vi "FA Bending View.vi"() -> ()   [LabVIEW 2016, in "M1M3SupportEUI_Views.lvlib"]
uses:
  M1M3SupportEUI_Views.lvlib
  Model/Model.lvclass
  M1M3 Support Events/M1M3 Support Events.lvclass/M1M3 Support Events.ctl
  SALLV_m1m3/DataTypes/command_ApplyAberrationForcesByBendingModes.ctl
  SALLV_m1m3/DataTypes/command_ClearAberrationForces.ctl
  SALLV_m1m3/DataTypes/command_ApplyActiveOpticForcesByBendingModes.ctl
  SALLV_m1m3/DataTypes/command_ClearActiveOpticForces.ctl
  M1M3 Support Events/M1M3 Support Events.lvclass
  SALLV_m1m3/SALLV_m1m3.lvlib
  EUI Events/EUI Events.lvclass
panel:
  in  "ClearActiveOpticsButton":bool
  in  "ApplyActiveOpticsByBendingModesButton":bool
  in  "ClearAberrationButton":bool
  in  "ApplyAberrationByBendingModesButton":bool
  in  "Model in":refnum<class "Model.lvclass">
  in  "BM1":sgl
  in  "BM2":sgl
  in  "BM3":sgl
  in  "BM4":sgl
  in  "BM5":sgl
  in  "BM6":sgl
  in  "BM7":sgl
  in  "BM8":sgl
  in  "BM9":sgl
  in  "BM20":sgl
  in  "BM10":sgl
  in  "BM12":sgl
  in  "BM13":sgl
  in  "BM14":sgl
  in  "BM15":sgl
  in  "BM16":sgl
  in  "BM17":sgl
  in  "BM18":sgl
  in  "BM19":sgl
  in  "BM11":sgl
  in  "BM22":sgl
  in  "BM21":sgl
  # "Force Actuator\nApply/Clear Bending Modes"
  # "Bending Modes"
  # "0"
  # "1"
  # "2"
  # "3"
  # "4"
  # "5"
  # "6"
  # "7"
  # "8"
  # "9"
  # "00"
  # "10"
  # "20"
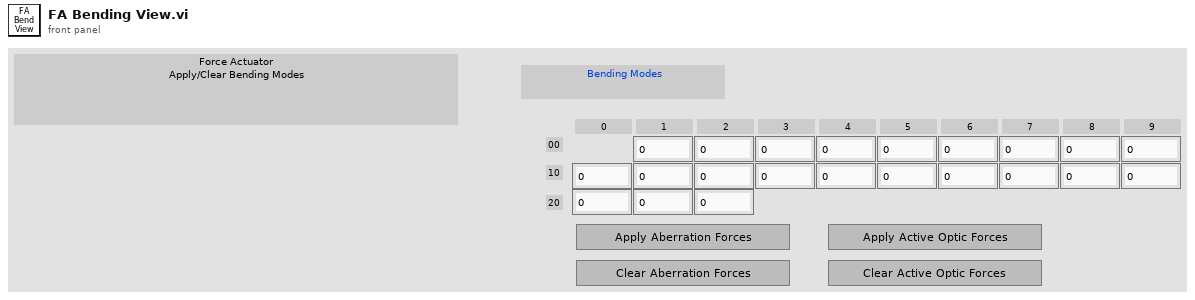
[diagram p1: front panel]
types:
  T1 = typedef "M1M3SupportEUI_TypeDefs.lvlib/M1M3 Support Events.ctl" = cluster{"Inclinometer  Data":refnum<user-event>, "IMS Data":refnum<user-event>, "SAL Connected":refnum<user-event>, "Accelerometer Data":refnum<user-event>, "OuterLoop Data":refnum<user-event>, "ErrorCode Event":refnum<user-event>, "InterlockStatus Event":refnum<user-event>, "InterlockWarning Event":refnum<user-event>, "Gyro Data":refnum<user-event>, "HP Actuator Info Event":refnum<user-event>, " FA Info Event":refnum<user-event>, "HP Monitor Info Event":refnum<user-event>, "FA Data":refnum<user-event>, "HP Actuator data":refnum<user-event>, "HP Monitor data":refnum<user-event>, "Air Supply Status Event":refnum<user-event>, "Air Supply Warning Event":refnum<user-event>, "Power Data":refnum<user-event>, "PID Data":refnum<user-event>, "PID Info Event":refnum<user-event>, "Power Status Event":refnum<user-event>, "Power Supply Status Event":refnum<user-event>, "Power Warning Event":refnum<user-event>, "Summary State Event":refnum<user-event>, "Detailed State Event":refnum<user-event>, "FA Force Warning Event":refnum<user-event>, "FA Warning Event":refnum<user-event>, "FA State Event":refnum<user-event>, "Applied AberrationForces Event":refnum<user-event>, "Applied Acceleration Forcces Event":refnum<user-event>, "Applied Azimuth Forces Event":refnum<user-event>, "Applied Active Optic Forces Event":refnum<user-event>, "Applied Balance Forces Event":refnum<user-event>, "Applied Cylinder Forces Event":refnum<user-event>, "Applied Elevation Forces Event":refnum<user-event>, "Applied Forces Event":refnum<user-event>, "Applied Offset Forces Event":refnum<user-event>, "Applied Static Forces Event":refnum<user-event>, "Applied Thermal Forces Event":refnum<user-event>, "Applied Velocity Forces Event":refnum<user-event>, "Rejected Aberration Force Event":refnum<user-event>, "Rejected Acceleration Forces Event":refnum<user-event>, "Rejected Active Optic Forces Event":refnum<user-event>, "Rejected Azimuth Forces Event":refnum<user-event>, "Rejected Balance Forces Event":refnum<user-event>, "Rejected Cylinder Forces Event":refnum<user-event>, "Rejected Elevation Forces Event":refnum<user-event>, "Rejected Forces Event":refnum<user-event>, "Rejected Offset Forces Event":refnum<user-event>, "Rejected Static Forces Event":refnum<user-event>, "Rejected Thermal Forces Event":refnum<user-event>, "Rejected Velocity Forces Event":refnum<user-event>, "Command Rejection Event":refnum<user-event>, "Setting Verions Event":refnum<user-event>, "Settings Applied Event":refnum<user-event>, "HP Actuator State Event":refnum<user-event>, "HP Actuator Warning Event":refnum<user-event>, "HP Monitor State Event":refnum<user-event>, "HP Monitor Warning Event":refnum<user-event>, "Accelerometer Warning Event":refnum<user-event>, "Applied Settings Match Start Event":refnum<user-event>, "Cell Light Status Event ":refnum<user-event>, "Cell Light Warning Event":refnum<user-event>, "Displacement Sensor Warning Event":refnum<user-event>, "Force Setpoint Warning Event":refnum<user-event>, "Gyro Warning Event ":refnum<user-event>, "ILC Warning Event ":refnum<user-event>, "Inclinometer Sensor Warning Event ":refnum<user-event>, "vms M1M3 Data":refnum<user-event>, "vms Acquisition Rate Event":refnum<user-event>, "vms Applied Settings Match Settings Event":refnum<user-event>, "vms Error Code Event":refnum<user-event>, "vms Setting Versions Event":refnum<user-event>, "vms Summary State Event":refnum<user-event>}
  T2 = enum16{"", "DetailedState_DetailedStates_DisabledState", "DetailedState_DetailedStates_EnabledState", "DetailedState_DetailedStates_FaultState", "DetailedState_DetailedStates_OfflineState", "DetailedState_DetailedStates_StandbyState", "DetailedState_DetailedStates_ParkedState", "DetailedState_DetailedStates_RaisingState", "DetailedState_DetailedStates_ActiveState", "DetailedState_DetailedStates_LoweringState", "DetailedState_DetailedStates_EngineeringState", "DetailedState_DetailedStates_ParkedEngineeringState", "DetailedState_DetailedStates_RaisingEngineeringState", "DetailedState_DetailedStates_ActiveEngineeringState", "DetailedState_DetailedStates_LoweringEngineeringState", "DetailedState_DetailedStates_LoweringFaultState", "DetailedState_DetailedStates_ProfileHardpointCorrectionState"}
  T3 = typedef "SALLV_m1m3.lvlib/command_ApplyAberrationForcesByBendingModes.ctl" = cluster{"Coefficients[22]":sgl[]}
  T4 = typedef "SALLV_m1m3.lvlib/command_ClearAberrationForces.ctl" = cluster{"ClearAberrationForces":bool}
  T5 = typedef "SALLV_m1m3.lvlib/command_ApplyActiveOpticForcesByBendingModes.ctl" = cluster{"Coefficients[22]":sgl[]}
  T6 = typedef "SALLV_m1m3.lvlib/command_ClearActiveOpticForces.ctl" = cluster{"ClearActiveOpticForces":bool}
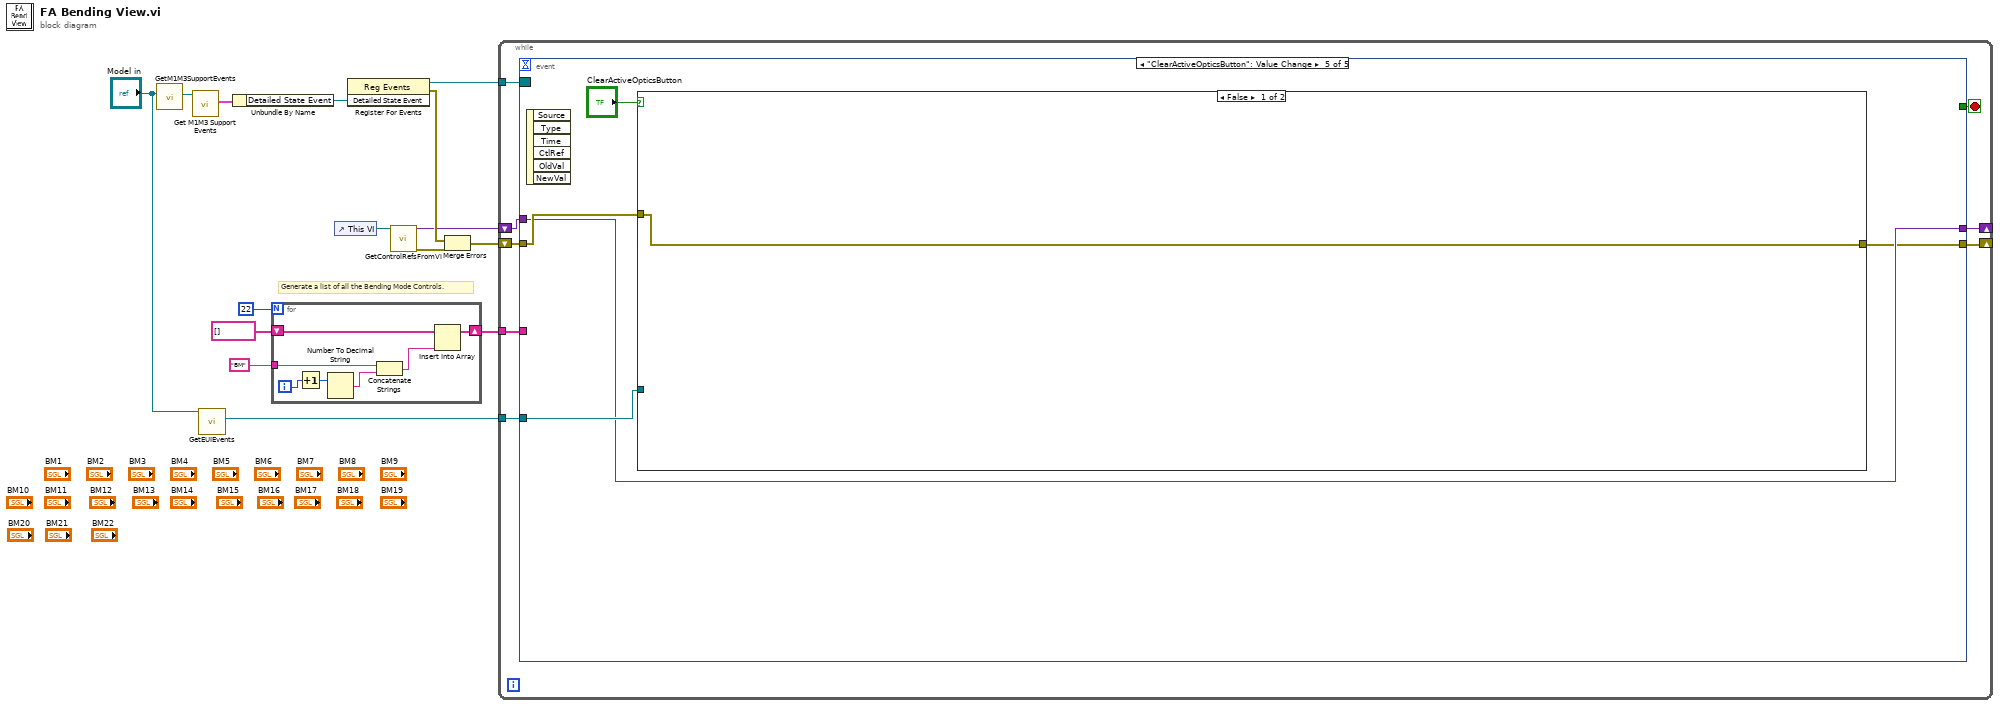
[diagram p0: block diagram]
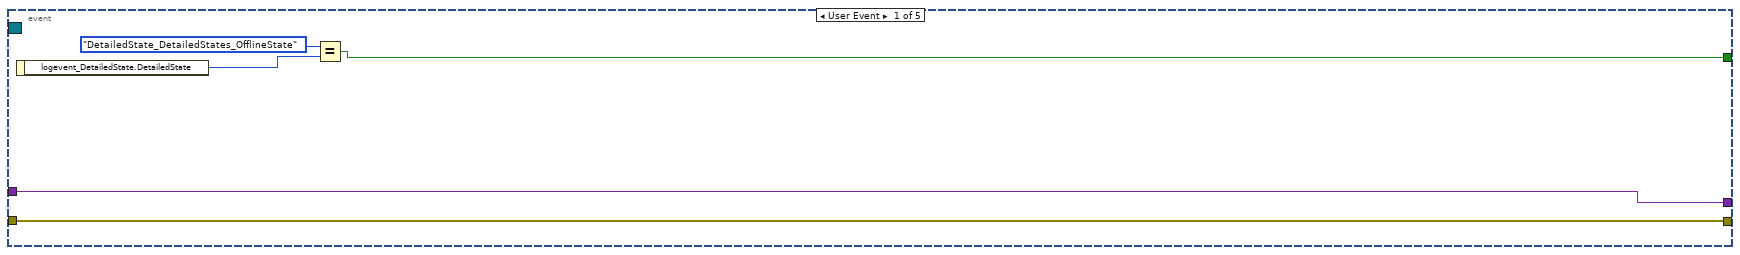
[diagram p2: hidden frame]
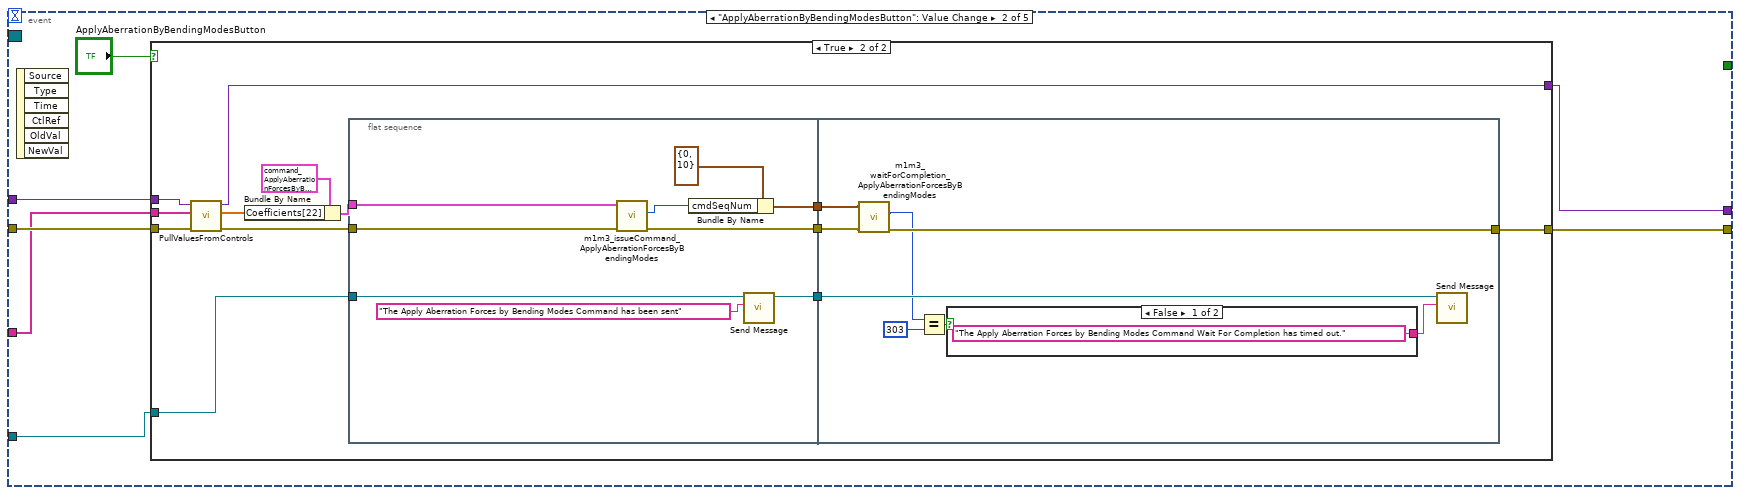
[diagram p3: hidden frame]
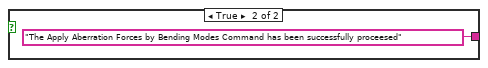
[diagram p5: hidden frame]
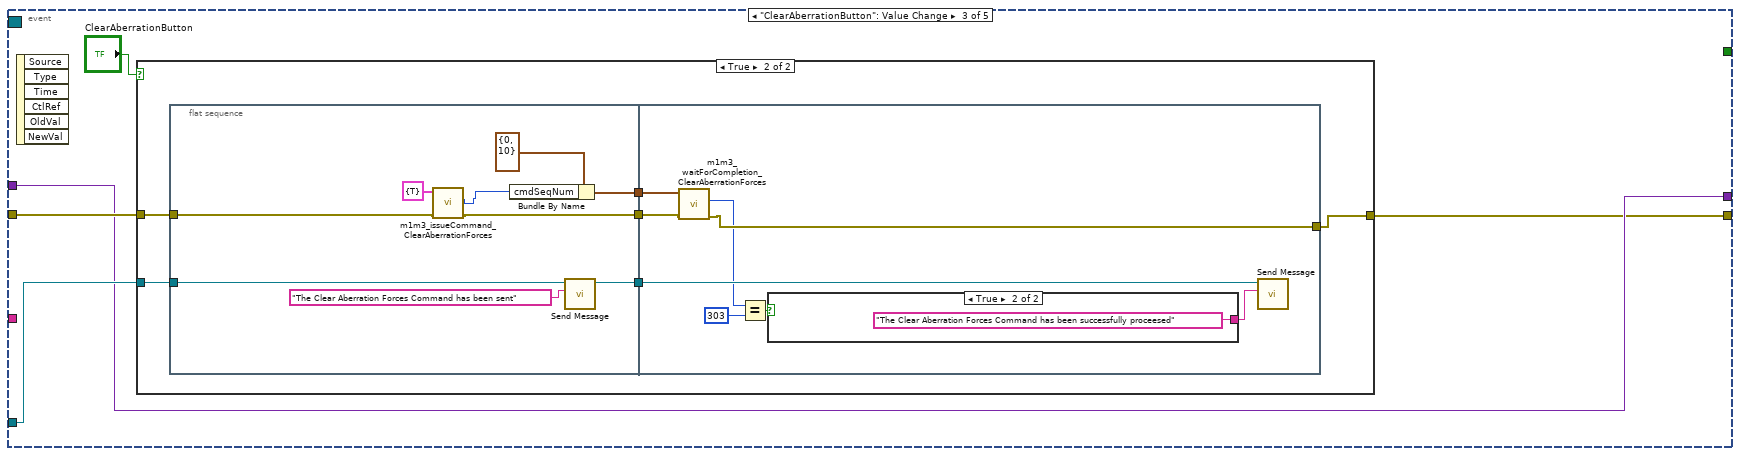
[diagram p6: hidden frame]
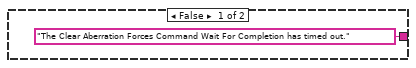
[diagram p8: hidden frame]
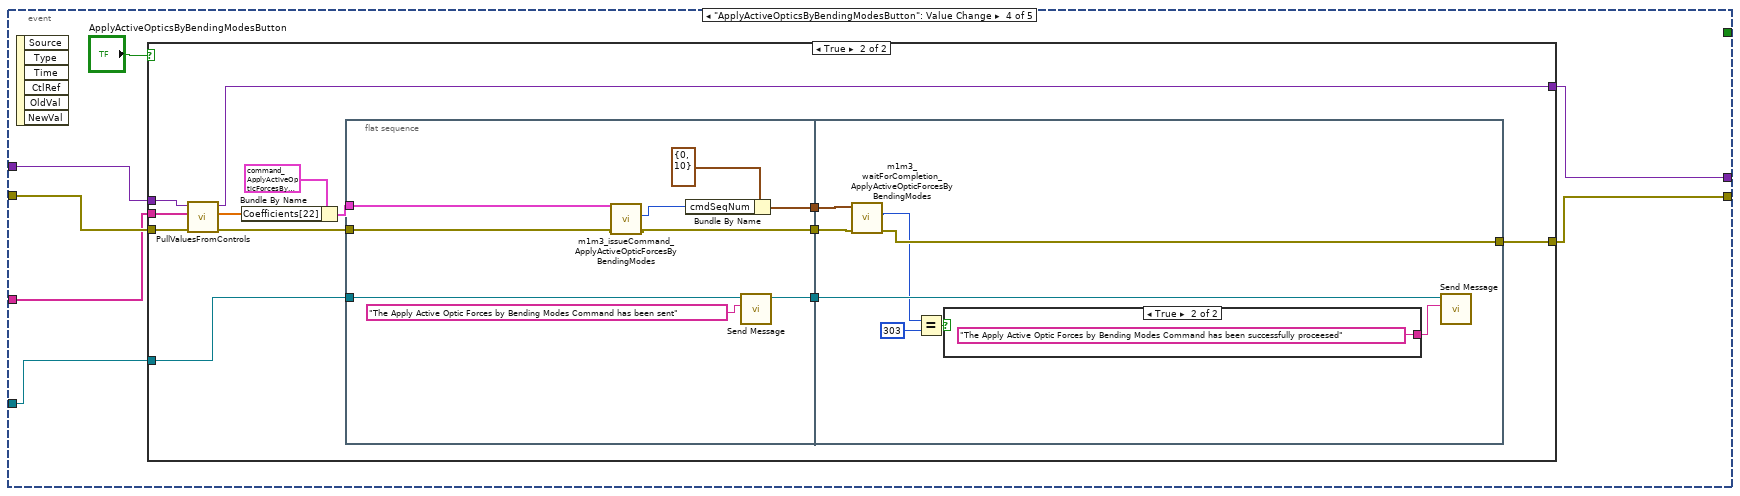
[diagram p9: hidden frame]
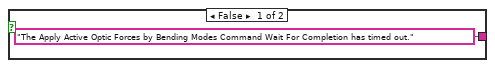
[diagram p11: hidden frame]
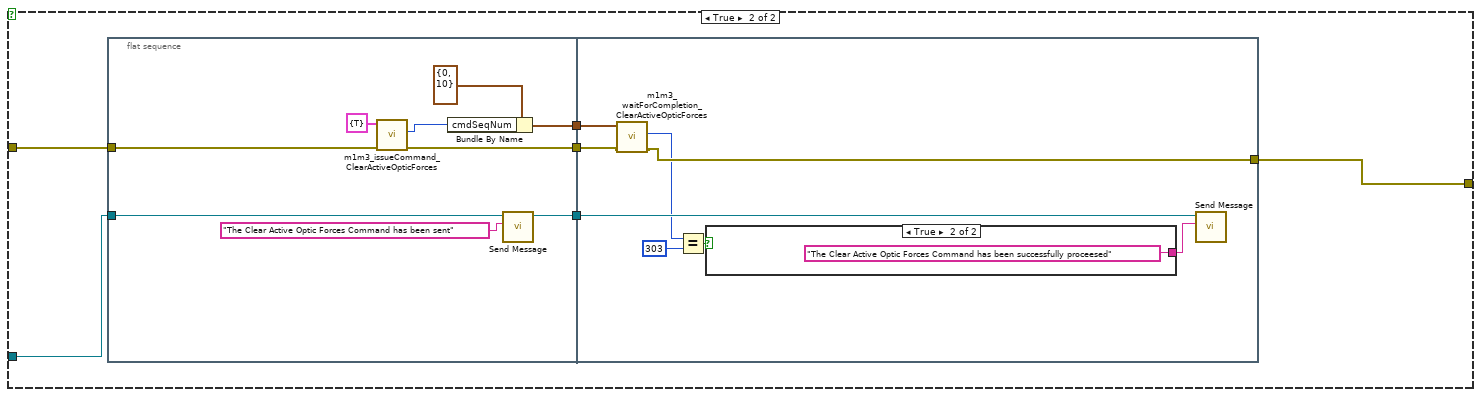
[diagram p12: hidden frame]
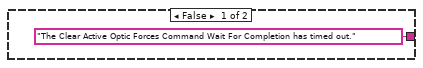
[diagram p13: hidden frame]
diagram:
  # "Generate a list of all the Bending Mode Controls."
  n1 = call "GetM1M3SupportEvents.vi"("Model in"="Model in") -> ("M1M3 Support Events out"=w14:refnum<class "M1M3 Support Events.lvclass">)  [unwired: 8 in, 2 out]
  n2 = call "Get M1M3 Support Events.vi"("M1M3 Support Events in"=w14) -> ("M1M3 Support Events"=w13:T1)  [unwired: 9 in, 1 out]
  n3 = call "GetEUIEvents.vi"("Model in"="Model in") -> ("EUI Events out"=w1:refnum<class "EUI Events.lvclass">)  [unwired: 8 in, 2 out]
  n4 = Unbundle By Name(w13) -> ("Detailed State Event"=w15:refnum<user-event>)
  n5 = for {
    N: 22 -> [_]
    shift-right: [w21] -> w3
    shift-left: string[] [] -> [w22]
    tunnel: "BM" -> [w20]
    i -> [w16]
    n6 = Increment(x=w16) -> (x+1=w17:i32)
    n7 = Number To Decimal String(number=w17) -> (decimal integer string=w19:string)  [unwired: 1 in]
    n8 = Concatenate Strings(w20, w19) -> (w18:string)
    n9 = Insert Into Array(array=w22, new element=w18) -> (w21:string[])  [unwired: 1 in]
  }
  n10 = control-ref of="This VI"() -> (w8:refnum<vi>)
  n11 = register-events(w15) -> (reference out=w9:refnum<event-registration>, error out=w6:errorcluster)  [unwired: 2 in]
  n12 = call "GetControlRefsFromVi.vi"("VI Refnum"=w8) -> ("error out"=w7:errorcluster, "Variant"=w4:variant)  [unwired: 9 in]
  n13 = Merge Errors(w6, w7) -> (w5:errorcluster)
  n14 = while {
    tunnel: w9 -> [w30]
    shift-right: [w23] -> _
    shift-left: w5 -> [w27]
    shift-right: [w24] -> _
    shift-left: w4 -> [w28]
    tunnel: w3 -> [w26]
    tunnel: w1 -> [w25]
    stop <- w29 stop-if-true
    n15 = event shown="[4] \"ClearActiveOpticsButton\": Value Change" {
      selector: w30 -> [_ _ _ _ _]
      dyn-events: _ -> [_ _ _ _ _]
      timeout: _ -> [_ _ _ _ _]
      tunnel: [w33 _ _ _ _] -> w29
      tunnel: w28 -> [w32 w41 w78 w113 w150]
      tunnel: w27 -> [w31 w40 w80 w112 w152]
      tunnel: w26 -> [_ w39 _ w111 _]
      tunnel: w25 -> [_ w38 w79 w110 w151]
      tunnel: [w32 w37 w78 w109 w150] -> w24
      tunnel: [w31 w36 w77 w108 w149] -> w23
      event User Event {
        n16 = event-data() -> ("logevent_DetailedState.DetailedState"=w35:T2)  [unwired: 1 in]
        n17 = Equal?(x=T2."DetailedState_DetailedStates_OfflineState", y=w35) -> (x = y?=w33:bool)
      }
      event "ApplyAberrationByBendingModesButton": Value Change {
        n18 = event-data() -> ()  [unwired: 1 in, 6 out]
        n19 = case shown="True" "ApplyAberrationByBendingModesButton" {
          tunnel: w41 -> [w43 w55]
          tunnel: w40 -> [w44 w54]
          tunnel: [w44 w51] -> w36
          tunnel: [w43 w48] -> w37
          tunnel: w39 -> [_ w47]
          tunnel: w38 -> [_ w46]
          frame False {
          }
          frame True {
            n20 = call "PullValuesFromControls.vi"("error in (no error)"=w54, "ControlNameArray"=w47, "Variant In"=w55) -> ("error out"=w53:errorcluster, "ControlValuesArray"=w56:sgl[], "Variant out"=w48:variant)  [unwired: 6 in]
            n21 = Bundle By Name(cluster=T3 {"Coefficients[22]"=[0.0, 0.0, 0.0, 0.0, 0.0, 0.0, 0.0, 0.0, 0.0, 0.0, 0.0, 0.0, 0.0, 0.0, 0.0, 0.0, 0.0, 0.0, 0.0, 0.0, 0.0, 0.0]} ("command_ApplyAberrationForcesByBendingModes"), "Coefficients[22]"=w56) -> (w50:T3)
            n22 = flat-sequence {
              tunnel: [w65] -> w57
              tunnel: w53 -> [w60]
              tunnel: [w58] -> w52
              tunnel: w50 -> [w61]
              tunnel: [w63] -> w49
              tunnel: w46 -> [w62]
              tunnel: w57 -> [w71]
              tunnel: w52 -> [w69]
              tunnel: [w68] -> w51
              tunnel: w49 -> [w70]
              frame #0 {
                n23 = call "m1m3_issueCommand_ApplyAberrationForcesByBendingModes.vi"("error in (no error)"=w60, "command_ApplyAberrationForcesByBendingModes_Ctl"=w61) -> ("error out"=w58:errorcluster, "function return"=w59:i32)  [unwired: 7 in, 1 out]
                n24 = Bundle By Name(cluster=cluster{"cmdSeqNum":i32, "timeout":u32} {"cmdSeqNum"=0, "timeout"=10} ("waitComplete_Ctl"), "cmdSeqNum"=w59) -> (w63:cluster{"cmdSeqNum":i32, "timeout":u32})
                n25 = call "Send Message.vi"("Message"="The Apply Aberration Forces by Bending Modes Command has been sent", "EUI Events in"=w62) -> ("EUI Events out"=w65:refnum<class "EUI Events.lvclass">)  [unwired: 8 in, 1 out]
              }
              frame #1 {
                n26 = call "m1m3_waitForCompletion_ApplyAberrationForcesByBendingModes.vi"("error in (no error)"=w69, "waitComplete_Ctl"=w70) -> ("error out"=w68:errorcluster, "function return"=w67:i32)  [unwired: 7 in, 1 out]
                n27 = Equal?(x=w67, y=303) -> (x = y?=w73:bool)
                n28 = case shown="False" w73 {
                  tunnel: ["The Apply Aberration Forces by Bending Modes Command Wait For Completion has timed out." ("Message") "The Apply Aberration Forces by Bending Modes Command has been successfully proceesed" ("Message")] -> w74
                  frame False {
                  }
                  frame True {
                  }
                }
                n29 = call "Send Message.vi"("Message"=w74, "EUI Events in"=w71) -> ()  [unwired: 8 in, 2 out]
              }
            }
          }
        }
      }
      event "ClearAberrationButton": Value Change {
        n30 = event-data() -> ()  [unwired: 1 in, 6 out]
        n31 = case shown="True" "ClearAberrationButton" {
          tunnel: w80 -> [w82 w85]
          tunnel: w79 -> [_ w84]
          tunnel: [w82 w83] -> w77
          frame False {
          }
          frame True {
            n32 = flat-sequence {
              tunnel: [w96] -> w88
              tunnel: w85 -> [w92]
              tunnel: [w91] -> w87
              tunnel: [w94] -> w86
              tunnel: w84 -> [w93]
              tunnel: w88 -> [w102]
              tunnel: w87 -> [w100]
              tunnel: [w99] -> w83
              tunnel: w86 -> [w101]
              frame #0 {
                n33 = call "m1m3_issueCommand_ClearAberrationForces.vi"("error in (no error)"=w92, "command_ClearAberrationForces_Ctl"=T4 {"ClearAberrationForces"=TRUE}) -> ("error out"=w91:errorcluster, "function return"=w90:i32)  [unwired: 7 in, 1 out]
                n34 = Bundle By Name(cluster=cluster{"cmdSeqNum":i32, "timeout":u32} {"cmdSeqNum"=0, "timeout"=10} ("waitComplete_Ctl"), "cmdSeqNum"=w90) -> (w94:cluster{"cmdSeqNum":i32, "timeout":u32})
                n35 = call "Send Message.vi"("Message"="The Clear Aberration Forces Command has been sent", "EUI Events in"=w93) -> ("EUI Events out"=w96:refnum<class "EUI Events.lvclass">)  [unwired: 8 in, 1 out]
              }
              frame #1 {
                n36 = call "m1m3_waitForCompletion_ClearAberrationForces.vi"("error in (no error)"=w100, "waitComplete_Ctl"=w101) -> ("error out"=w99:errorcluster, "function return"=w98:i32)  [unwired: 7 in, 1 out]
                n37 = Equal?(x=w98, y=303) -> (x = y?=w104:bool)
                n38 = case shown="True" w104 {
                  tunnel: ["The Clear Aberration Forces Command Wait For Completion has timed out." ("Message") "The Clear Aberration Forces Command has been successfully proceesed" ("Message")] -> w105
                  frame False {
                  }
                  frame True {
                  }
                }
                n39 = call "Send Message.vi"("Message"=w105, "EUI Events in"=w102) -> ()  [unwired: 8 in, 2 out]
              }
            }
          }
        }
      }
      event "ApplyActiveOpticsByBendingModesButton": Value Change {
        n40 = event-data() -> ()  [unwired: 1 in, 6 out]
        n41 = case shown="True" "ApplyActiveOpticsByBendingModesButton" {
          tunnel: w113 -> [w115 w127]
          tunnel: w112 -> [w116 w126]
          tunnel: [w116 w123] -> w108
          tunnel: [w115 w120] -> w109
          tunnel: w111 -> [_ w119]
          tunnel: w110 -> [_ w118]
          frame False {
          }
          frame True {
            n42 = call "PullValuesFromControls.vi"("error in (no error)"=w126, "ControlNameArray"=w119, "Variant In"=w127) -> ("error out"=w125:errorcluster, "ControlValuesArray"=w128:sgl[], "Variant out"=w120:variant)  [unwired: 6 in]
            n43 = Bundle By Name(cluster=T5 {"Coefficients[22]"=[0.0, 0.0, 0.0, 0.0, 0.0, 0.0, 0.0, 0.0, 0.0, 0.0, 0.0, 0.0, 0.0, 0.0, 0.0, 0.0, 0.0, 0.0, 0.0, 0.0, 0.0, 0.0]} ("command_ApplyActiveOpticForcesByBendingModes"), "Coefficients[22]"=w128) -> (w122:T5)
            n44 = flat-sequence {
              tunnel: [w137] -> w129
              tunnel: w125 -> [w131]
              tunnel: [w133] -> w124
              tunnel: w122 -> [w130]
              tunnel: [w135] -> w121
              tunnel: w118 -> [w134]
              tunnel: w129 -> [w143]
              tunnel: w124 -> [w139]
              tunnel: [w141] -> w123
              tunnel: w121 -> [w142]
              frame #0 {
                n45 = call "m1m3_issueCommand_ApplyActiveOpticForcesByBendingModes.vi"("error in (no error)"=w131, "command_ApplyActiveOpticForcesByBendingModes_Ctl"=w130) -> ("error out"=w133:errorcluster, "function return"=w132:i32)  [unwired: 7 in, 1 out]
                n46 = Bundle By Name(cluster=cluster{"cmdSeqNum":i32, "timeout":u32} {"cmdSeqNum"=0, "timeout"=10} ("waitComplete_Ctl"), "cmdSeqNum"=w132) -> (w135:cluster{"cmdSeqNum":i32, "timeout":u32})
                n47 = call "Send Message.vi"("Message"="The Apply Active Optic Forces by Bending Modes Command has been sent", "EUI Events in"=w134) -> ("EUI Events out"=w137:refnum<class "EUI Events.lvclass">)  [unwired: 8 in, 1 out]
              }
              frame #1 {
                n48 = call "m1m3_waitForCompletion_ApplyActiveOpticForcesByBendingModes.vi"("error in (no error)"=w139, "waitComplete_Ctl"=w142) -> ("error out"=w141:errorcluster, "function return"=w140:i32)  [unwired: 7 in, 1 out]
                n49 = Equal?(x=w140, y=303) -> (x = y?=w145:bool)
                n50 = case shown="True" w145 {
                  tunnel: ["The Apply Active Optic Forces by Bending Modes Command Wait For Completion has timed out." ("Message") "The Apply Active Optic Forces by Bending Modes Command has been successfully proceesed" ("Message")] -> w146
                  frame False {
                  }
                  frame True {
                  }
                }
                n51 = call "Send Message.vi"("Message"=w146, "EUI Events in"=w143) -> ()  [unwired: 8 in, 2 out]
              }
            }
          }
        }
      }
      event "ClearActiveOpticsButton": Value Change {
        n52 = event-data() -> ()  [unwired: 1 in, 6 out]
        n53 = case shown="False" "ClearActiveOpticsButton" {
          tunnel: w152 -> [w154 w157]
          tunnel: w151 -> [_ w156]
          tunnel: [w154 w155] -> w149
          frame False {
          }
          frame True {
            n54 = flat-sequence {
              tunnel: [w168] -> w160
              tunnel: w157 -> [w164]
              tunnel: [w163] -> w159
              tunnel: [w166] -> w158
              tunnel: w156 -> [w165]
              tunnel: w160 -> [w174]
              tunnel: w159 -> [w172]
              tunnel: [w171] -> w155
              tunnel: w158 -> [w173]
              frame #0 {
                n55 = call "m1m3_issueCommand_ClearActiveOpticForces.vi"("error in (no error)"=w164, "command_ClearActiveOpticForces_Ctl"=T6 {"ClearActiveOpticForces"=TRUE}) -> ("error out"=w163:errorcluster, "function return"=w162:i32)  [unwired: 7 in, 1 out]
                n56 = Bundle By Name(cluster=cluster{"cmdSeqNum":i32, "timeout":u32} {"cmdSeqNum"=0, "timeout"=10} ("waitComplete_Ctl"), "cmdSeqNum"=w162) -> (w166:cluster{"cmdSeqNum":i32, "timeout":u32})
                n57 = call "Send Message.vi"("Message"="The Clear Active Optic Forces Command has been sent", "EUI Events in"=w165) -> ("EUI Events out"=w168:refnum<class "EUI Events.lvclass">)  [unwired: 8 in, 1 out]
              }
              frame #1 {
                n58 = call "m1m3_waitForCompletion_ClearActiveOpticForces.vi"("error in (no error)"=w172, "waitComplete_Ctl"=w173) -> ("error out"=w171:errorcluster, "function return"=w170:i32)  [unwired: 7 in, 1 out]
                n59 = Equal?(x=w170, y=303) -> (x = y?=w176:bool)
                n60 = case shown="True" w176 {
                  tunnel: ["The Clear Active Optic Forces Command Wait For Completion has timed out." ("Message") "The Clear Active Optic Forces Command has been successfully proceesed" ("Message")] -> w177
                  frame False {
                  }
                  frame True {
                  }
                }
                n61 = call "Send Message.vi"("Message"=w177, "EUI Events in"=w174) -> ()  [unwired: 8 in, 2 out]
              }
            }
          }
        }
      }
    }
  }
